vi "PMTprocess.vi"(11 "PMT Settings":cluster{"Bin Length":dbl, "Show Mean":bool}) -> (3 "PMT":dbl[][](graph))   [LabVIEW 2017]
uses:
  <vilib>/rvi/interface/nirviReadWriteControl/nirviReadWriteControl.xnode
  <vilib>/Analysis/NI_AALBase.lvlib
  <vilib>/Analysis/baseanly.llb/Mean (DBL).vi
  NiFpgaLv.dll
  <vilib>/Utility/error.llb/Error Cluster From Error Code.vi
  <vilib>/rvi/interface/Simulation/niFpgaSimulationCallBeginRW.vi
  <vilib>/rvi/errors/niLvFpgaAdjustHostInterfaceError.vi
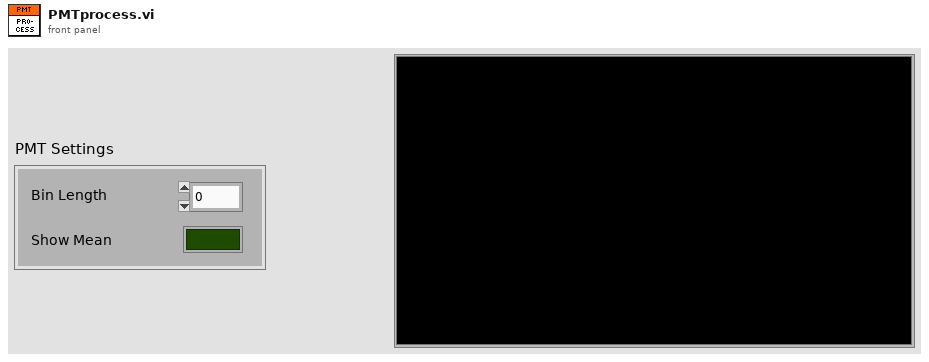
[diagram p1: front panel]
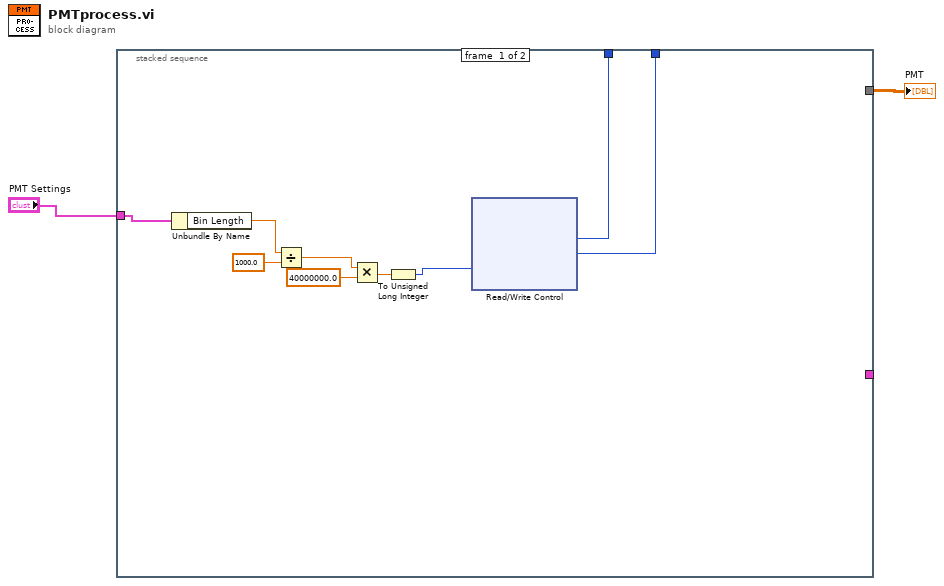
[diagram p0: block diagram]
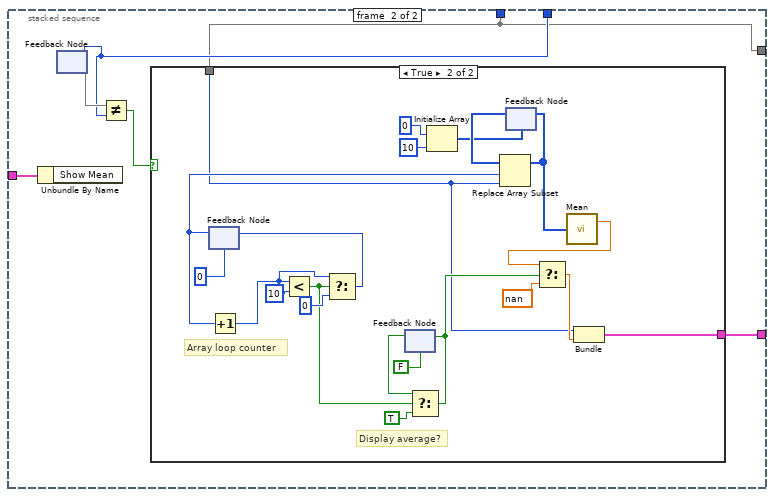
[diagram p2: hidden frame]
diagram:
  n1 = stacked-sequence {
    tunnel: "PMT Settings" -> [w11 w16]
    tunnel: [w4 w12] -> _
    tunnel: [w3 w14] -> _
    tunnel: [_ w15] -> _
    tunnel: "PMT" -> [_ w12]
    frame #0 {
      n2 = Unbundle By Name(w11) -> ("Bin Length"=w7:dbl)
      n3 = Divide(x=w7, y=1000.0) -> (x/y=w9:dbl)
      n4 = Multiply(x=w9, y=40000000.0) -> (x*y=w6:dbl)
      n5 = To Unsigned Long Integer(number=w6) -> (unsigned 32bit integer=w5:u32)
      n6 = xnode "Read/Write Control"("ticks per bin"=w5) -> ("Frequency Chart"=w4:u32, "bin number"=w3:u32)  [unwired: 2 in, 4 out]
    }
    frame #1 {
      n7 = Unbundle By Name(w16) -> ()  [unwired: 1 out]
      n8 = feedback #1() -> (w17)  [unwired: 1 in]
      n9 = feedback-in #1(w14) -> ()
      n10 = Not Equal?(x=w17, y=w14) -> (x != y?=w13:bool)
      n11 = case shown="True" w13 {
        tunnel: [_ w19] -> w15
        tunnel: [_ w18] -> w12
        frame False {
        }
        frame True {
          # "Display average?"
          # "Array loop counter"
          n12 = feedback #2(0) -> (w21:i32)
          n13 = Increment(x=w21) -> (x+1=w37:i32)
          n14 = Less?(x=w37, y=10) -> (x < y?=w29:bool)
          n15 = Select(t=w37, s=w29, f=0) -> (s? t:f=w20:i32)
          n16 = feedback-in #2(w20) -> ()
          n17 = feedback #3(FALSE) -> (w23:bool)
          n18 = Select(t=w23, s=w29, f=TRUE) -> (s? t:f=w22:bool)
          n19 = feedback-in #3(w22) -> ()
          n20 = Initialize Array(u32 0 ("Frequency Chart"), 10 ("dimension size")) -> (w31:u32[])
          n21 = feedback #4(w31) -> (w34:u32[])
          n22 = Replace Array Subset(array=w34, index=w21) -> (w30:u32[], new element=w18:u32)
          n23 = feedback-in #4(w30) -> ()
          n24 = call-poly <vilib>:"Mean.vi"("X"=w30) -> ("mean"=w25:dbl)  [unwired: 1 out]
          n25 = Select(t=w25, s=w22, f=nan) -> (s? t:f=w26:dbl)
          n26 = Bundle(w18, "f"=w26) -> (w19:cluster{void, "f":dbl})  [unwired: 1 in]
        }
      }
    }
  }
